vi "Set Fields.vi"(8 "error in":errorcluster, 10 "Fields":variant[](array[variant]), 11 "Info Section in":refnum<class "Info Section.lvclass">) -> (0 "error out":errorcluster, 3 "Info Section out":refnum<class "Info Section.lvclass">)   [LabVIEW 2025, in "Electronic Datasheet.lvlib" / "Info Section.lvclass"]
uses:
  Info Section.lvclass
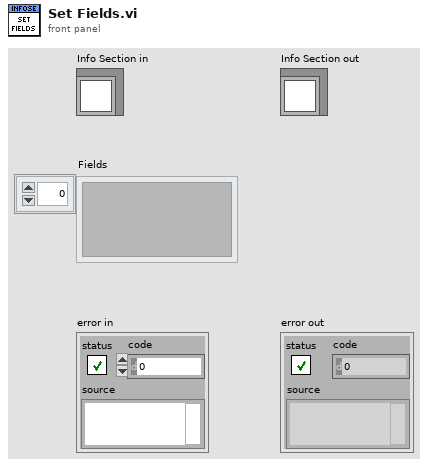
[diagram p1: front panel]
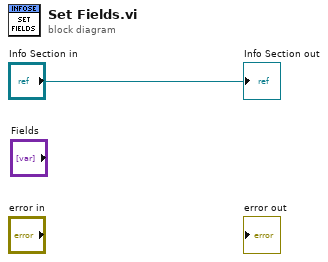
[diagram p0: block diagram]
diagram:
  "Info Section out" <- "Info Section in"
